vi "Close.vi"(8 "error in (no error)":errorcluster, 11 "SMP in":refnum<class "SMP.lvclass">) -> (0 "error out":errorcluster)   [LabVIEW 2013, in "SMP.lvclass"]
doc: "Closes the input SMP object."
uses:
  SMP.lvclass
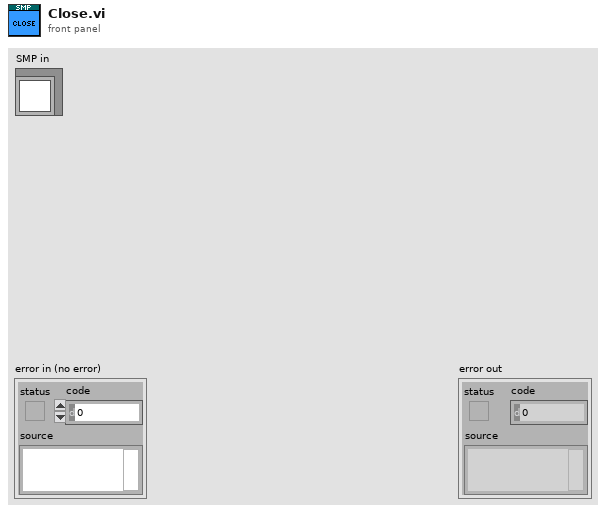
[diagram p1: front panel]
types:
  T1 = typedef "Pipe and Filter.lvclass/classData.ctl" = cluster{"Q ref":refnum<queue>, "Previous data":variant, "Current pipe":T2[]}
  T2 = typedef "Pipe and Filter.lvclass/operation.ctl" = cluster{"Name":string, "Data":variant}
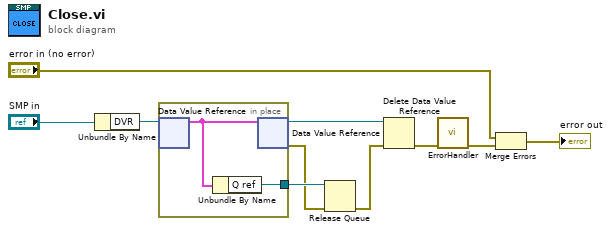
[diagram p0: block diagram]
diagram:
  n1 = Unbundle By Name("SMP in") -> ("DVR"=w8:refnum<data-value>)
  n2 = in-place {
    in-place-border: [w11] -> w7
    n3 = in-place-dvr #1(w8) -> (w12:T1)  [unwired: 1 out]
    n4 = Unbundle By Name(w12) -> ("Q ref"=w11:refnum<queue>)
    n5 = in-place-dvr #1(w12) -> (w5:refnum<data-value>, w6:errorcluster)
  }
  n6 = Release Queue(queue=w7, error in (no error)=w6) -> (error out=w4:errorcluster)  [unwired: 1 in, 2 out]
  n7 = Delete Data Value Reference(data value reference=w5, error in=w4) -> (error out=w3:errorcluster)  [unwired: 1 out]
  n8 = call "ErrorHandler.vi"("error in (no error)"=w3) -> ("error out"=w10:errorcluster)  [unwired: 9 in, 1 out]
  n9 = Merge Errors("error in (no error)", w10) -> (→"error out":errorcluster)
